vi "ke37xx Configure Relative Control.vi"(0 "VISA Resource Name":refnum<visa-resource-name>, 5 "Relative Control Enabled (F: Disabled)":bool, 7 "Relative Level (0)":dbl=0.02, 11 "error in (no error)":errorcluster) -> (4 "VISA Resource Name Out":refnum<visa-resource-name>, 15 "error out":errorcluster)   [LabVIEW 2009, in "Keithley 3700 Series.lvlib"]
doc: "This VI allows you to control the relative measurement capabiliteis of the DMM. When relative measurements are enabled, all subsequent measured readings will be offset by the specified relative offset. Specifically, each returned measured relative reading will be the result of the the following calculation:\n\nRelative Reading = Actual Measured Reading - Relative Offset Value"
uses:
  <instrlib>/Keithley 3706/Keithley 3700 Series.lvlib
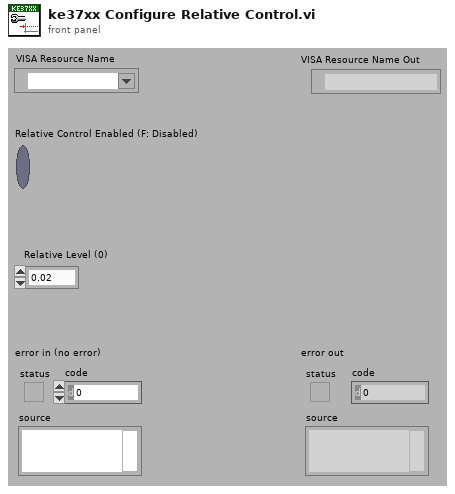
[diagram p1: front panel]
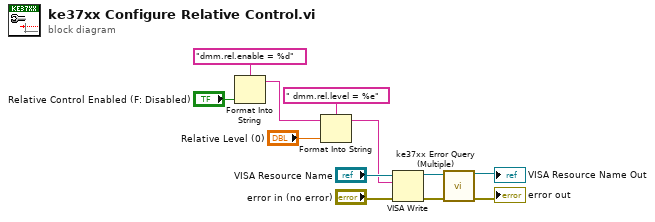
[diagram p0: block diagram]
diagram:
  n1 = Format Into String(format string="dmm.rel.enable = %d" ("write buffer"), "Relative Control Enabled (F: Disabled)") -> (resulting string=w2:string)  [unwired: 2 in, 1 out]
  n2 = Format Into String(format string=" dmm.rel.level = %e" ("write buffer"), initial string=w2, "Relative Level (0)") -> (resulting string=w5:string)  [unwired: 1 in, 1 out]
  n3 = VISA Write(VISA resource name="VISA Resource Name", write buffer=w5, error in (no error)="error in (no error)") -> (VISA resource name out=w8:refnum<visa-resource-name>, error out=w7:errorcluster)  [unwired: 1 out]
  n4 = call <instrlib>:"ke37xx Error Query (Multiple).vi"("VISA resource name"=w8, "error in (no error)"=w7) -> ("VISA resource name out"=→"VISA Resource Name Out":refnum<visa-resource-name>, "error out"=→"error out":errorcluster)  [unwired: 12 out]
